vi "PSA Marker Search.vi"(8 "error in (no error)":errorcluster, 9 "Mark Search":u16(ring) items=["Highest", "Next Peak", "Next Peak Left", "Next Peak Right", "Minimum", "Pk-Pk Search"], 10 "Active Marker":u16(ring)=1 items=["Marker1"=1, "Marker2"=2, "Marker3"=3, "Marker4"=4], 11 "VISA resource name":refnum<visa-resource-name>) -> (0 "error out":errorcluster, 3 "VISA resource name out":refnum<visa-resource-name>)   [LabVIEW 2014]
uses:
  Agilent ESA PSA Series.lvlib
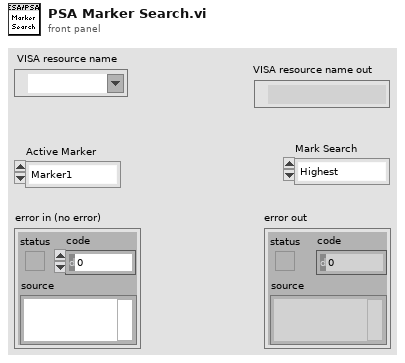
[diagram p1: front panel]
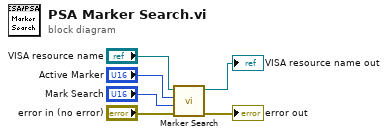
[diagram p0: block diagram]
diagram:
  n1 = call "Marker Search.vi"("error in (no error)"="error in (no error)", "Mark Search (0: Highest)"="Mark Search", "Active Marker (1: Marker1)"="Active Marker", "VISA resource name"="VISA resource name") -> ("error out"=→"error out":errorcluster, "VISA resource name out"=→"VISA resource name out":refnum<visa-resource-name>)  [unwired: 6 in]
